vi "check_config_file_presence.vi"(6 "progress slider":refnum<vi>, 8 "error in (no error)":errorcluster, 11 "steps":T1[](array[typedef])) -> (0 "error out":errorcluster, 3 "present?":bool[](array[boolean]))   [LabVIEW 2010]
uses:
  common/clusters/plugin_specification.ctl
  common/classes/GenericComponent/GenericComponent/GenericComponent.lvclass
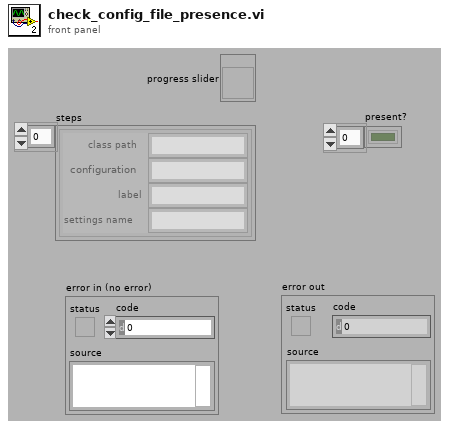
[diagram p1: front panel]
types:
  T1 = typedef "plugin_specification.ctl" = cluster{"class path":string, "configuration":string, "label":string, "settings name":string}
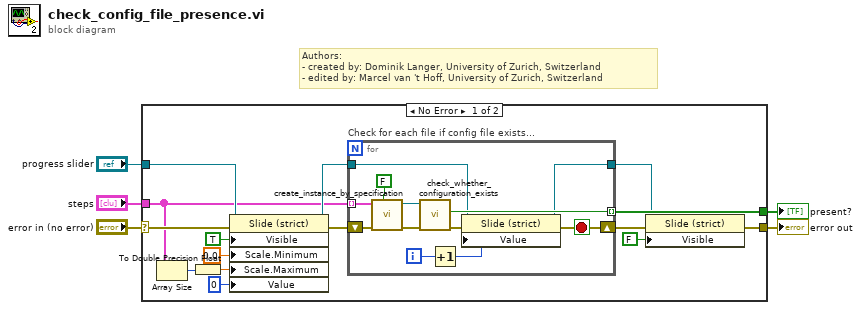
[diagram p0: block diagram]
diagram:
  # "Authors: \n- created by: Dominik Langer, University of Zurich, Switzerland\n- edited by: Marcel van 't Hoff, University of Zurich, Switzerland"
  n1 = case shown="No Error" "error in (no error)" {
    selector: "error in (no error)" -> [w18 w33]
    tunnel: "steps" -> [w10 _]
    tunnel: [w13 w33] -> w4
    tunnel: [w20 _] -> w3
    tunnel: "progress slider" -> [w19 _]
    frame No Error {
      n2 = Array Size(array=w10) -> (size(s)=w9:i32)
      n3 = To Double Precision Float(number=w9) -> (double precision float=w8:dbl)
      n4 = property class="Slide (strict)"(reference=w19, error in=w18, "Visible"=TRUE, "Scale.Minimum"=0.0 ("Scale.Range:Minimum"), "Scale.Maximum"=w8, "Value"=0) -> (reference out=w15:refnum<vi>, error out=w17:errorcluster)
      n5 = for "Check for each file if config file exists..." {
        tunnel: [w27] -> w20 mode=indexing
        tunnel: w10 -> [w30] mode=indexing
        shift-right: [w21] -> w14
        shift-left: w17 -> [w31]
        tunnel: [w23] -> w6
        tunnel: w15 -> [w24]
        i -> [w26]
        stop <- w21 stop-if-true
        n6 = call "create_instance_by_specification.vi"("call constructor?"=FALSE, "error in (no error)"=w31, "component specification"=w30) -> ("error out"=w29:errorcluster, "GenericPlugin out"=w28:refnum<class "GenericComponent.lvclass">)  [unwired: 6 in, 1 out]
        n7 = call-dynamic "check_whether_configuration_exists.vi"("error in (no error)"=w29, "GenericPlugin in"=w28) -> ("error out"=w22:errorcluster, "exists?"=w27:bool)  [unwired: 7 in, 1 out]
        n8 = Increment(x=w26) -> (x+1=w25:i32)
        n9 = property class="Slide (strict)"(reference=w24, error in=w22, "Value"=w25) -> (reference out=w23:refnum<vi>, error out=w21:errorcluster)
      }
      n10 = property class="Slide (strict)"(reference=w6, error in=w14, "Visible"=FALSE) -> (error out=w13:errorcluster)  [unwired: 1 out]
    }
    frame Error {
    }
  }
  "error out" <- w4
  "present?" <- w3
